vi "Init Alarm MSGs.vi"(8 "error in (no error)":errorcluster) -> (0 "error out":errorcluster)   [LabVIEW 2020]
uses:
  PCT FGV CMD.ctl
  <vilib>/Utility/file.llb/Read Delimited Spreadsheet (string).vi
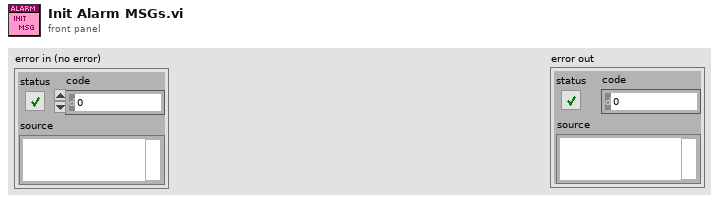
[diagram p1: front panel]
types:
  T1 = typedef "PCT FGV CMD.ctl" = enum16{"INIT", "GET", "SET"}
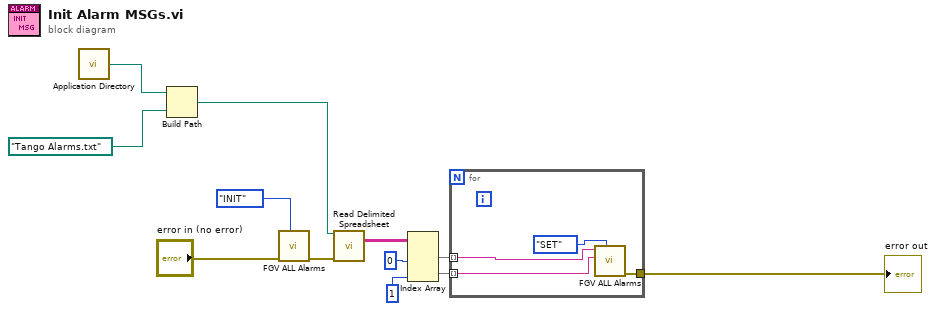
[diagram p0: block diagram]
diagram:
  n1 = call <vilib>:"Application Directory.vi"() -> ("Application Directory"=w5:path)
  n2 = Build Path(base path=w5, name or relative path=path "Tango Alarms.txt" ("file path (dialog if empty)")) -> (appended path=w1:path)
  n3 = call "FGV ALL Alarms.vi"("CMD"=PCT_FGV_CMD."INIT", "error in (no error)"="error in (no error)") -> ("error out"=w9:errorcluster)  [unwired: 8 in, 1 out]
  n4 = call-poly <vilib>:"Read Delimited Spreadsheet.vi"("file path (dialog if empty)"=w1, "error in (no error)"=w9) -> ("all rows"=w12:string[][])  [unwired: 8 in, 5 out]
  n5 = Index Array(array=w12, index (col) #1=0 ("disabled index (col)"), index (col) #2=1 ("disabled index (col)")) -> (element #1=w11:string[], element #2=w2:string[])  [unwired: 2 in]
  n6 = for {
    tunnel: w11 -> [w14] mode=indexing
    tunnel: [w15] -> w7
    tunnel: w2 -> [w13] mode=indexing
    n7 = call "FGV ALL Alarms.vi"("CMD"=PCT_FGV_CMD."SET", "Alarm MSG in"=w13, "name"=w14) -> ("error out"=w15:errorcluster)  [unwired: 7 in, 1 out]
  }
  "error out" <- w7
